vi "SaveCsv.vi"(0 "path":path=path "D:/Database", 1 "所有测试数据":string[][](array[string])=[["SN", "NA", "NA", "NA", "NA", "NA", "NA", "NA", "NA", ""], ["AC(mA)", "54", "42", "654", "354", "34", "543", "25", "45", ""], ["IR(Mohm)", "54", "42", "654", "354", "34", "543", "25", "45", ""], ["Result", "PASS", "FAIL", "PASS", "FAIL", "PASS", "FAIL", "FAIL", "FAIL", ""], ["", "", "", "", "", "", "", "", "", "NA"]], 2 "File_Name":string) -> ()   [LabVIEW 2018]
uses:
  Subvi/Global.vi
  <vilib>/Utility/file.llb/Write Delimited Spreadsheet (string).vi
panel:
  out "数组 4":string[][](array[string])
  out "数组 3":string[][](array[string])
  out "添加的路径":path
  out "数组 2":string[][](array[string])
  out "子数组":string[](array[string])
  out "数组":string[][](array[string])
  out "所有测试数据 2":string[][](array[string])
  out "大小":i32[](array[numeric])
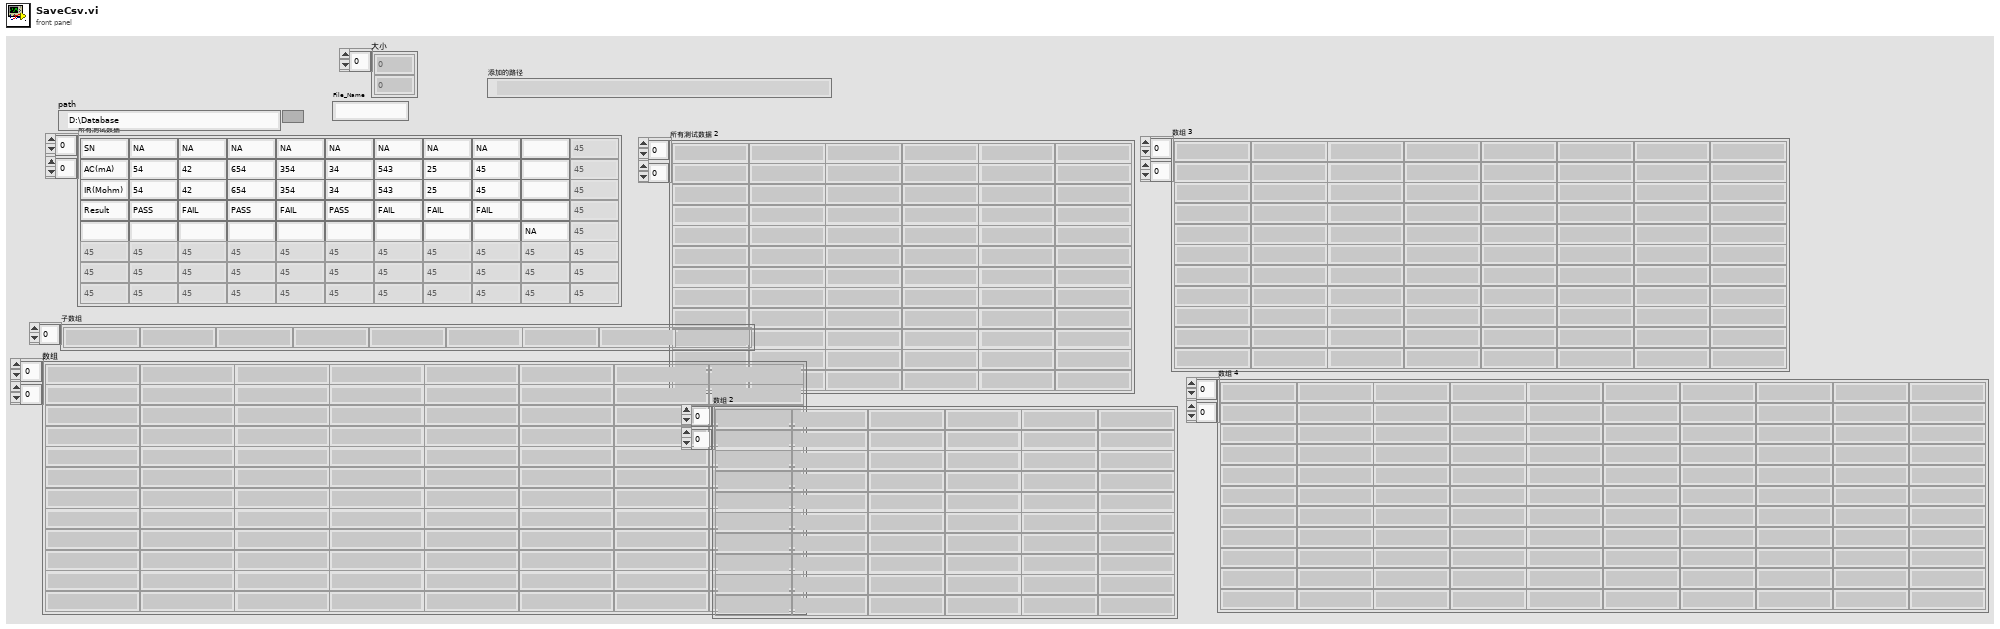
[diagram p1: front panel]
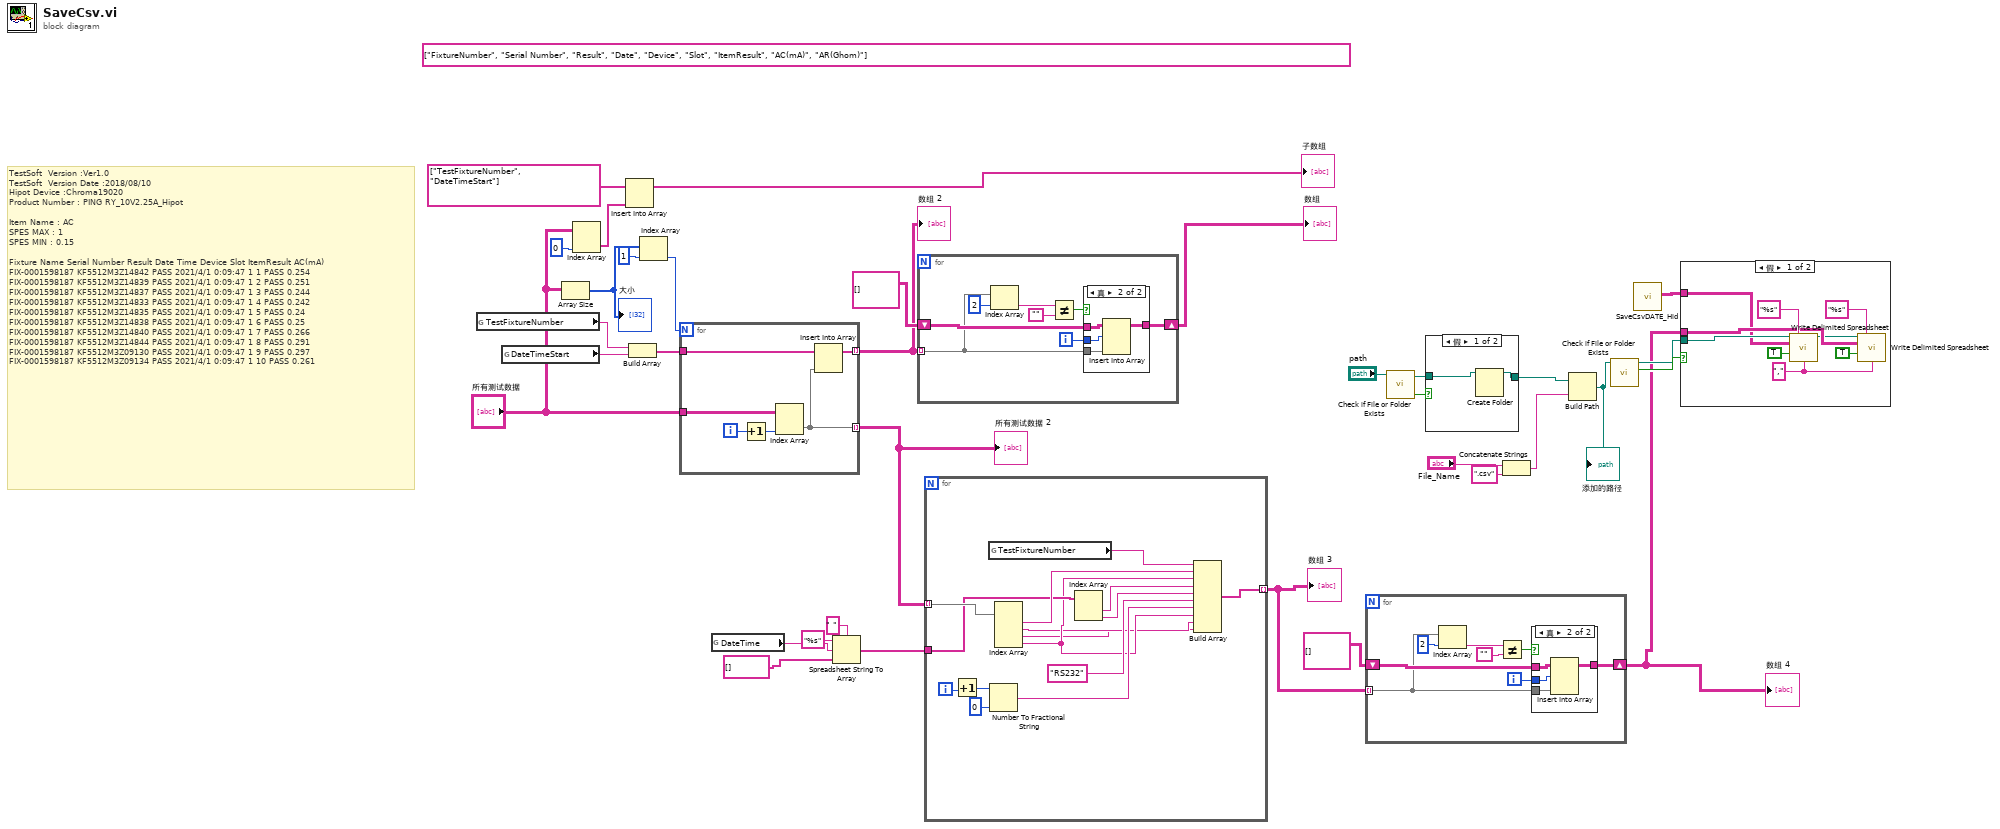
[diagram p0: block diagram]
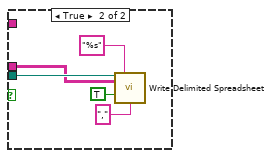
[diagram p4: hidden frame]
diagram:
  (unwired) string[] ["FixtureNumber", "Serial Number", "Result", "Date", "Device", "Slot", "ItemResult", "AC(mA)", "AR(Ghom)"]
  # "TestSoft  Version :Ver1.0\t\t\t\t\t\t\t\t\nTestSoft  Version Date :2018/08/10\t\t\t\t\t\t\t\t\nHipot Device :Chroma19020\t\t\t\t\t\t\t\t\nProduct Number :\tPING RY_10V2.25A_Hipot\t\t\t\t\t\t\t\n\t\t\t\t\t\t\t\t\nItem Name :\tAC\t\t\t\t\t\t\t\nSPES MAX :\t1\t\t\t\t\t\t\t\nSPES MIN :\t0.15\t\t\t\t\t\t\t\n\t\t\t\t\t\t\t\t\nFixture Name\tSerial Number\tResult\tDate\tTime\tDevice\tSlot\tItemResult\tAC(mA)\nFIX-0001598187\tKF5512M3Z14842\tPASS\t2021/4/1\t0:09:47\t1\t1\tPASS\t0.254\nFIX-0001598187\tKF5512M3Z14839\tPASS\t2021/4/1\t0:09:47\t1\t2\tPASS\t0.251\nFIX-0001598187\tKF5512M3Z14837\tPASS\t2021/4/1\t0:09:47\t1\t3\tPASS\t0.244\nFIX-0001598187\tKF5512M3Z14833\tPASS\t2021/4/1\t0:09:47\t1\t4\tPASS\t0.242\nFIX-0001598187\tKF5512M3Z14835\tPASS\t2021/4/1\t0:09:47\t1\t5\tPASS\t0.24\nFIX-0001598187\tKF5512M3Z14838\tPASS\t2021/4/1\t0:09:47\t1\t6\tPASS\t0.25\nFIX-0001598187\tKF5512M3Z14840\tPASS\t2021/4/1\t0:09:47\t1\t7\tPASS\t0.266\nFIX-0001598187\tKF5512M3Z14844\tPASS\t2021/4/1\t0:09:47\t1\t8\tPASS\t0.291\nFIX-0001598187\tKF5512M3Z09130\tPASS\t2021/4/1\t0:09:47\t1\t9\tPASS\t0.297\nFIX-0001598187\tKF5512M3Z09134\tPASS\t2021/4/1\t0:09:47\t1\t10\tPASS\t0.261"
  n1 = global read "Global.vi" "TestFixtureNumber"() -> (w31:string)
  n2 = global read "Global.vi" "DateTimeStart"() -> (w26:string)
  n3 = Array Size(array="所有测试数据") -> (size(s)=w34:i32[])
  "大小" <- w34
  n4 = Index Array(array="所有测试数据", index (col)=0 ("禁用的索引 (列)")) -> (element=w27:string[])  [unwired: 1 in]
  n5 = Insert Into Array(array=string[] ["TestFixtureNumber", "DateTimeStart"], new element=w27) -> (→"子数组":string[])  [unwired: 1 in]
  n6 = Build Array(w31, w26) -> (w30:string[])
  n7 = Index Array(array=w34, index=1 ("索引")) -> (element=w33:i32)
  n8 = for {
    N: w33 -> [_]
    tunnel: "所有测试数据" -> [w37]
    tunnel: [w39] -> w9 mode=indexing
    tunnel: w30 -> [w40]
    tunnel: [w38] -> w23 mode=indexing
    i -> [w36]
    n9 = Increment(x=w36) -> (x+1=w35:i32)
    n10 = Index Array(array=w37, index (col)=w35) -> (element=w39:string[])  [unwired: 1 in]
    n11 = Insert Into Array(array=w40, new element=w39) -> (w38:string[])  [unwired: 1 in]
  }
  "所有测试数据 2" <- w9
  "数组 2" <- w23
  n12 = global read "Global.vi" "DateTime"() -> (w5:string)
  n13 = Spreadsheet String To Array(delimiter (Tab)=" " ("分隔符(Tab)"), format string="%s" ("格式字符串"), spreadsheet string=w5, array type (2D Dbl)=string[] []) -> (array=w4:string[])
  n14 = for {
    shift-right: [w47] -> w20
    shift-left: string[][] [] -> [w48]
    tunnel: w23 -> [w41] mode=indexing
    i -> [w46]
    n15 = Index Array(array=w41, index=2 ("索引")) -> (element=w44:string)
    n16 = Not Equal?(x=w44, y="") -> (x != y?=w42:bool)
    n17 = case shown="真" w42 {
      tunnel: w48 -> [w49 w53]
      tunnel: [w49 w52] -> w47
      tunnel: w46 -> [_ w51]
      tunnel: w41 -> [_ w50]
      frame False {
      }
      frame True {
        n18 = Insert Into Array(array=w53, index (row)=w51, new element=w50) -> (w52:string[][])  [unwired: 1 in]
      }
    }
  }
  "数组" <- w20
  n19 = for {
    tunnel: w9 -> [w68] mode=indexing
    tunnel: w4 -> [w62]
    tunnel: [w56] -> w2 mode=indexing
    i -> [w67]
    n20 = Increment(x=w67) -> (x+1=w66:i32)
    n21 = global read "Global.vi" "TestFixtureNumber"() -> (w64:string)
    n22 = Number To Fractional String(number=w66, precision (6)=i16 0 ("精度(6)")) -> (F-format string=w58:string)  [unwired: 2 in]
    n23 = Index Array(array=w68) -> (element #1=w63:string, element #2=w55:string, element #3=w54:string, element #4=w57:string)  [unwired: 4 in]
    n24 = Index Array(array=w62) -> (element #1=w61:string, element #2=w60:string)  [unwired: 2 in]
    n25 = Build Array(w64, w63, w57, w61, w60, "RS232", w58, w57, w55, w54) -> (w56:string[])
  }
  "数组 3" <- w2
  n26 = for {
    shift-right: [w75] -> w1
    shift-left: string[][] [] -> [w76]
    tunnel: w2 -> [w69] mode=indexing
    i -> [w74]
    n27 = Index Array(array=w69, index=2 ("索引")) -> (element=w72:string)
    n28 = Not Equal?(x=w72, y="") -> (x != y?=w70:bool)
    n29 = case shown="真" w70 {
      tunnel: w76 -> [w77 w81]
      tunnel: [w77 w80] -> w75
      tunnel: w74 -> [_ w79]
      tunnel: w69 -> [_ w78]
      frame False {
      }
      frame True {
        n30 = Insert Into Array(array=w81, index (row)=w79, new element=w78) -> (w80:string[][])  [unwired: 1 in]
      }
    }
  }
  "数组 4" <- w1
  n31 = call <vilib>:"Check if File or Folder Exists.vi"("path"="path") -> ("file or folder exists?"=w17:bool, "dup path"=w16:path)  [unwired: 8 in, 1 out]
  n32 = case shown="假" w17 {
    tunnel: w16 -> [w83 w84]
    tunnel: [w82 w84] -> w15
    frame False {
      n33 = Create Folder(path (use dialog)=w83) -> (created path=w82:path)  [unwired: 2 in, 2 out]
    }
    frame True {
    }
  }
  n34 = Concatenate Strings("File_Name", ".csv") -> (w11:string)
  n35 = Build Path(base path=w15, name or relative path=w11) -> (appended path=w14:path)
  "添加的路径" <- w14
  n36 = call <vilib>:"Check if File or Folder Exists.vi"("path"=w14) -> ("file or folder exists?"=w22:bool, "dup path"=w21:path)  [unwired: 8 in, 1 out]
  n37 = call "SaveCsvDATE_Hid.vi"() -> ("输出数组"=w10:string[][])  [unwired: 11 in]
  n38 = case shown="假" w22 {
    tunnel: w21 -> [w91 w98]
    tunnel: w1 -> [w90 w97]
    tunnel: w10 -> [w85 _]
    frame False {
      w87 = "," ("delimiter (\\t)")
      n39 = call-poly <vilib>:"Write Delimited Spreadsheet.vi"("file path (dialog if empty)"=w91, "format (%s)"="%s", "2D data"=w85, "append to file? (new file:F)"=TRUE, "delimiter (\\t)"=w87) -> ("new file path (Not A Path if cancelled)"=w89:path)  [unwired: 9 in, 1 out]
      n40 = call-poly <vilib>:"Write Delimited Spreadsheet.vi"("file path (dialog if empty)"=w89, "format (%s)"="%s", "2D data"=w90, "append to file? (new file:F)"=TRUE, "delimiter (\\t)"=w87) -> ()  [unwired: 9 in, 2 out]
    }
    frame True {
      n41 = call-poly <vilib>:"Write Delimited Spreadsheet.vi"("file path (dialog if empty)"=w98, "format (%s)"="%s", "2D data"=w97, "append to file? (new file:F)"=TRUE, "delimiter (\\t)"="," ("delimiter (\\t)")) -> ()  [unwired: 9 in, 2 out]
    }
  }
